vi "Method One Numeric Argument.vi"(8 "error in (no error)":errorcluster, 10 "Numeric":dbl, 11 "Test Interface Mock In":refnum<class "Test Interface Pure Mock.lvclass">) -> (0 "error out":errorcluster, 3 "Test Interface Mock Out":refnum<class "Test Interface Pure Mock.lvclass">)   [LabVIEW 2020, in "Test Interface Pure Mock.lvclass"]
uses:
  Test Interface Pure Mock.lvclass
  C:/git/astemes-lmock/source/Framework/Pure Mock/Pure Mock.lvclass
  source/Framework/Pure Mock/Pure Mock.lvclass/Pure Mock.ctl
  source/Framework/Parametric VI Call/Parametric VI Call.lvclass
  C:/git/astemes-lmock/source/Core/VI Call/VI Call.lvclass
  source/Framework/Parametric VI Call/Create.vi
  source/Core/Expectation/Expectation.lvclass
  source/Framework/Pure Mock/Pure Mock.lvclass
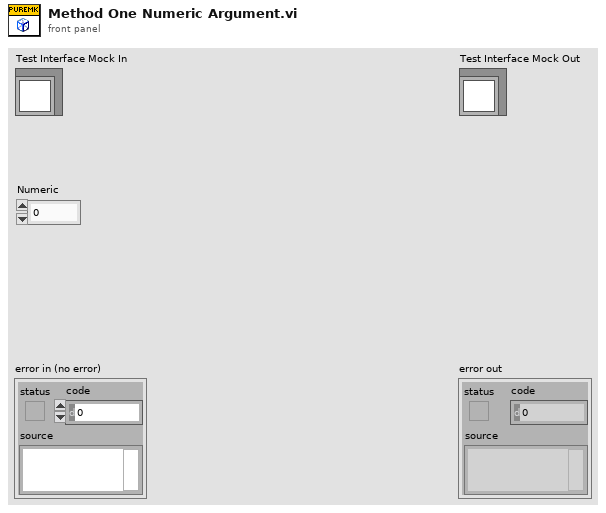
[diagram p1: front panel]
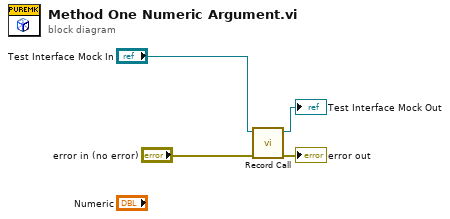
[diagram p0: block diagram]
diagram:
  n1 = call "Record Call.vi"("error in (no error)"="error in (no error)", "Mock In"="Test Interface Mock In") -> ("error out"=→"error out":errorcluster, "Mock Out"=→"Test Interface Mock Out":refnum<class "Test Interface Pure Mock.lvclass">)  [unwired: 8 in]
